vi "Capture Stopped.vi"(8 "error in (no error)":errorcluster, 11 "Camera_Controller in":refnum<class "Camera_Controller.lvclass">) -> (0 "error out":errorcluster, 3 "Camera_Controller out":refnum<class "Camera_Controller.lvclass">)   [LabVIEW 2023, in "CameraLibrary.lvlib" / "Camera_Controller.lvlib" / "Camera_Controller.lvclass"]
uses:
  Camera_Controller.lvclass
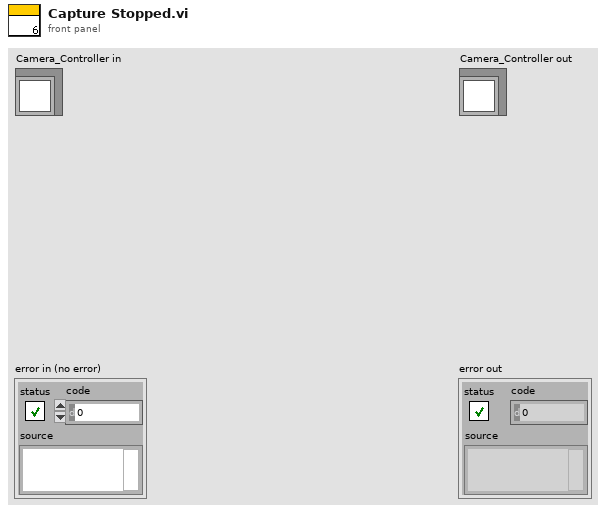
[diagram p1: front panel]
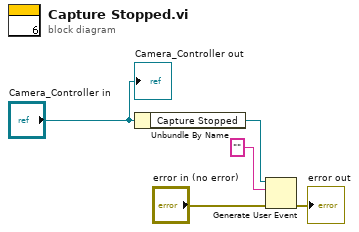
[diagram p0: block diagram]
diagram:
  n1 = Unbundle By Name("Camera_Controller in") -> ("Capture Stopped"=w2:refnum<user-event>)
  n2 = Generate User Event(user event=w2, event data cluster="" ("event data"), error in="error in (no error)") -> (error out=→"error out":errorcluster)  [unwired: 1 in, 1 out]
  "Camera_Controller out" <- "Camera_Controller in"
